vi "(SubVI) Calculate Xbd and Xst for pFC_YCC.vi"(4 "Target QPD radius (nm)":dbl=500.0, 6 "Target QPD (V)":dbl, 7 "cr":dbl, 8 "X=T\nY=F":bool=TRUE, 9 "Stage Position":dbl[](array[numeric]), 10 "QPD signal":dbl[](array[numeric]), 11 "conversion factor (V/um)":dbl=1.0) -> (2 "Xst (nm)":dbl[](array[numeric]), 3 "Xbd (nm)":dbl[](array[numeric]))   [LabVIEW 2014]
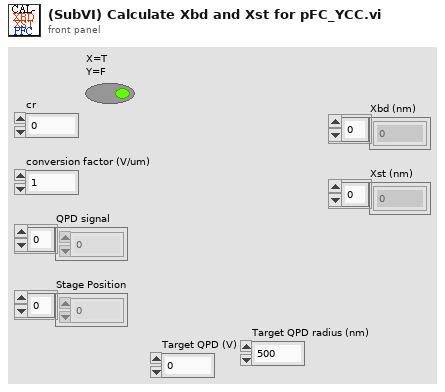
[diagram p1: front panel]
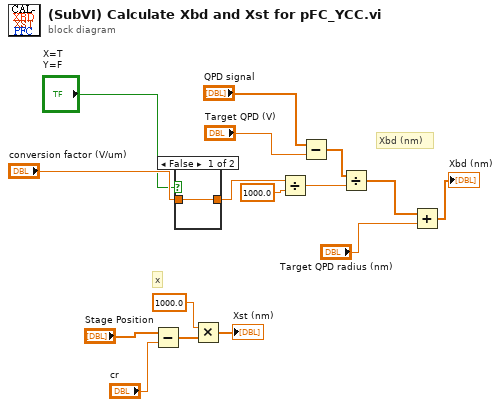
[diagram p0: block diagram]
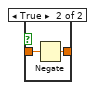
[diagram p2: hidden frame]
diagram:
  # "x"
  # "Xbd (nm)"
  n1 = Subtract(x="Stage Position", y="cr") -> (x-y=w8:dbl[])
  n2 = case shown="False" "X=T\nY=F" {
    tunnel: "conversion factor (V/um)" -> [w17 w19]
    tunnel: [w17 w18] -> w5
    frame False {
    }
    frame True {
      n3 = Negate(x=w19) -> (-x=w18:dbl)
    }
  }
  n4 = Multiply(x=1000.0, y=w8) -> (x*y=→"Xst (nm)":dbl[])
  n5 = Divide(x=w5, y=1000.0) -> (x/y=w15:dbl)
  n6 = Subtract(x="QPD signal", y="Target QPD (V)") -> (x-y=w7:dbl[])
  n7 = Divide(x=w7, y=w15) -> (x/y=w3:dbl[])
  n8 = Add(x=w3, y="Target QPD radius (nm)") -> (x+y=→"Xbd (nm)":dbl[])
